vi "_Engine Core.vi"(11 "Engine Control":T1) -> ()   [LabVIEW 2013]
uses:
  EngineControl.ctl
  <vilib>/Utility/miscctls.llb/LVPositionTypeDef.ctl
  Move Speed.ctl
  Positioning Strategy.ctl
panel:
  out "Numeric":i32
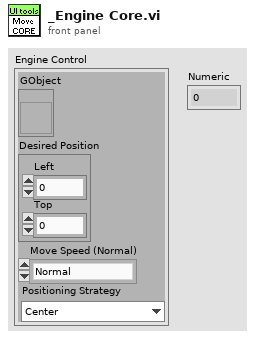
[diagram p1: front panel]
types:
  T1 = typedef "EngineControl.ctl" = cluster{"GObject":refnum<vi>, "Desired Position":T2, "Move Speed (Normal)":T3, "Positioning Strategy":T4}
  T2 = typedef "LVPositionTypeDef.ctl" = cluster{"Left":i32, "Top":i32}
  T3 = typedef "Move Speed.ctl" = enum16{"Normal", "Fast", "Slow", "Instantaneous"}
  T4 = typedef "Positioning Strategy.ctl" = enum16{"Center", "Origin (Top-Left)"}
  T5 = typedef "LVBoundsTypeDef.ctl" = cluster{"Width":u32, "Height":u32}
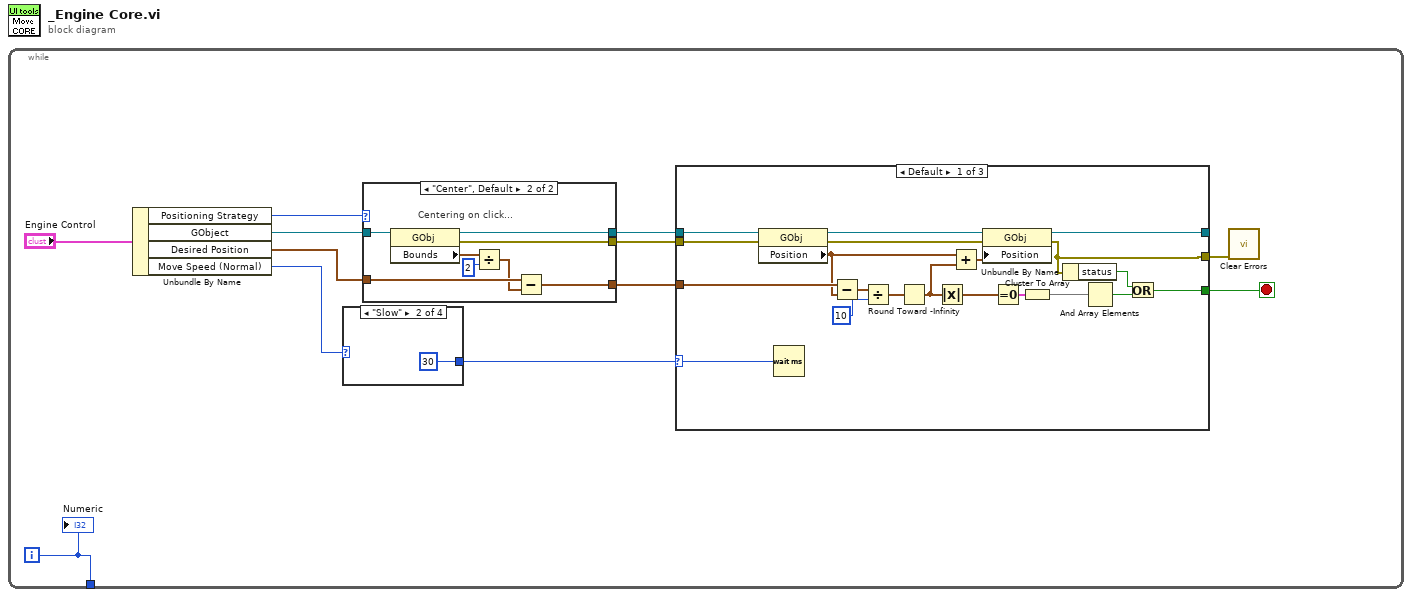
[diagram p0: block diagram]
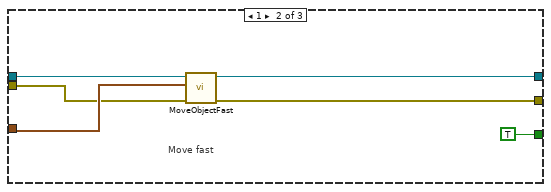
[diagram p3: hidden frame]
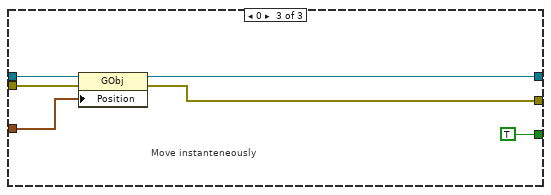
[diagram p4: hidden frame]
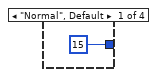
[diagram p5: hidden frame]
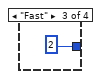
[diagram p6: hidden frame]
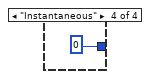
[diagram p7: hidden frame]
diagram:
  n1 = while {
    tunnel: [w2] -> _
    i -> [w2]
    stop <- w3 stop-if-true
    n2 = Unbundle By Name("Engine Control") -> ("Positioning Strategy"=w1:T4, "GObject"=w11:refnum<vi>, "Desired Position"=w10:T2, "Move Speed (Normal)"=w9:T3)
    n3 = case shown="\"Slow\"" w9 {
      tunnel: [u32 15 ("Sliding Speed (40)") u32 30 ("Sliding Speed (40)") u32 2 ("Sliding Speed (40)") u32 0 ("Sliding Speed (40)")] -> w6
      frame "Normal", Default {
      }
      frame "Slow" {
      }
      frame "Fast" {
      }
      frame "Instantaneous" {
      }
    }
    n4 = case shown="\"Center\", Default" w1 {
      tunnel: w11 -> [w13 w22]
      tunnel: w10 -> [w14 w21]
      tunnel: [w13 w20] -> w8
      tunnel: [_ w19] -> w7
      tunnel: [w14 w15] -> w4
      frame "Origin (Top-Left)" {
      }
      frame "Center", Default {
        # "Centering on click..."
        n5 = property class="GObj"(reference=w22) -> (reference out=w20:refnum<vi>, error out=w19:errorcluster, "Bounds"=w18:T5)  [unwired: 1 in]
        n6 = Divide(x=w18, y=2) -> (x/y=w16:cluster{"Width":dbl, "Height":dbl})
        n7 = Subtract(x=w21, y=w16) -> (x-y=w15:cluster{dbl, dbl})
      }
    }
    n8 = case shown="Default" w6 {
      selector: w6 -> [w38 _ _]
      tunnel: w8 -> [w42 w48 w52]
      tunnel: w7 -> [w41 w46 w53]
      tunnel: w4 -> [w40 w47 w51]
      tunnel: [w39 w45 w54] -> _
      tunnel: [w37 w44 w50] -> w5
      tunnel: [w36 TRUE TRUE] -> w3
      frame Default {
        n9 = property class="GObj"(reference=w42, error in=w41) -> (reference out=w35:refnum<vi>, error out=w29:errorcluster, "Position"=w32:T2)
        n10 = Wait (ms)(milliseconds to wait=w38) -> ()  [unwired: 1 out]
        n11 = Subtract(x=w40, y=w32) -> (x-y=w31:cluster{"Left":dbl, "Top":dbl})
        n12 = Divide(x=w31, y=10) -> (x/y=w25:cluster{"Left":dbl, "Top":dbl})
        n13 = Round Toward -Infinity(1:w25) -> (0:w24:cluster{"Left":dbl, "Top":dbl})
        n14 = Absolute Value(x=w24) -> (abs(x)=w23:cluster{"Left":dbl, "Top":dbl})
        n15 = Add(x=w32, y=w24) -> (x+y=w26:cluster{"Left":dbl, "Top":dbl})
        n16 = property class="GObj"(reference=w35, error in=w29, "Position"=w26) -> (reference out=w39:refnum<vi>, error out=w37:errorcluster)
        n17 = Equal To 0?(x=w23) -> (x = 0?=w33:cluster{"Left":bool, "Top":bool})
        n18 = Cluster To Array(cluster=w33) -> (array=w34:bool[])
        n19 = Unbundle By Name(w37) -> ("status"=w27:bool)
        n20 = And Array Elements(Boolean array=w34) -> (logical AND=w28:bool)
        n21 = Or(x=w27, y=w28) -> (x .or. y?=w36:bool)
      }
      frame 1 {
        # "Move fast"
        n22 = call "MoveObjectFast.vi"("error in"=w46, "Position"=w47, "GObj Refnum"=w48) -> ("error out"=w44:errorcluster, "GObj Refnum dup"=w45:refnum<vi>)  [unwired: 7 out]
      }
      frame 0 {
        # "Move instanteneously"
        n23 = property class="GObj"(reference=w52, error in=w53, "Position"=w51) -> (reference out=w54:refnum<vi>, error out=w50:errorcluster)
      }
    }
    n24 = call <vilib>:"Clear Errors.vi"("error in (no error)"=w5) -> ()  [unwired: 7 out]
    "Numeric" <- w2
  }
